vi "Draw_multiple_lines.vi"() -> ()   [LabVIEW 2023]
panel:
  in  "Actualizar":bool
  in  "String":string
  in  "Bobina":T1={"pen"={"Width"=1, "Style"=enum."Solid"}, "color(black)"=0, "fill?(F)"=FALSE, "line endpoints"=[]}
  in  "Resistencia 2":T2={"line endpoints"=[], "pen"={"Width"=1, "Style"=enum."Solid"}, "color(black)"=0, "fill?(F)"=FALSE}
  in  "Fuente":T3={"line endpoints"=[], "pen"={"Width"=1, "Style"=enum."Solid"}, "color(black)"=0, "fill?(F)"=FALSE, "line endpoints 2"=[]}
  in  "Capacitor":T3={"line endpoints"=[], "pen"={"Width"=1, "Style"=enum."Solid"}, "color(black)"=0, "fill?(F)"=FALSE, "line endpoints 2"=[]}
  out "new picture":picture
  in  "stop":bool
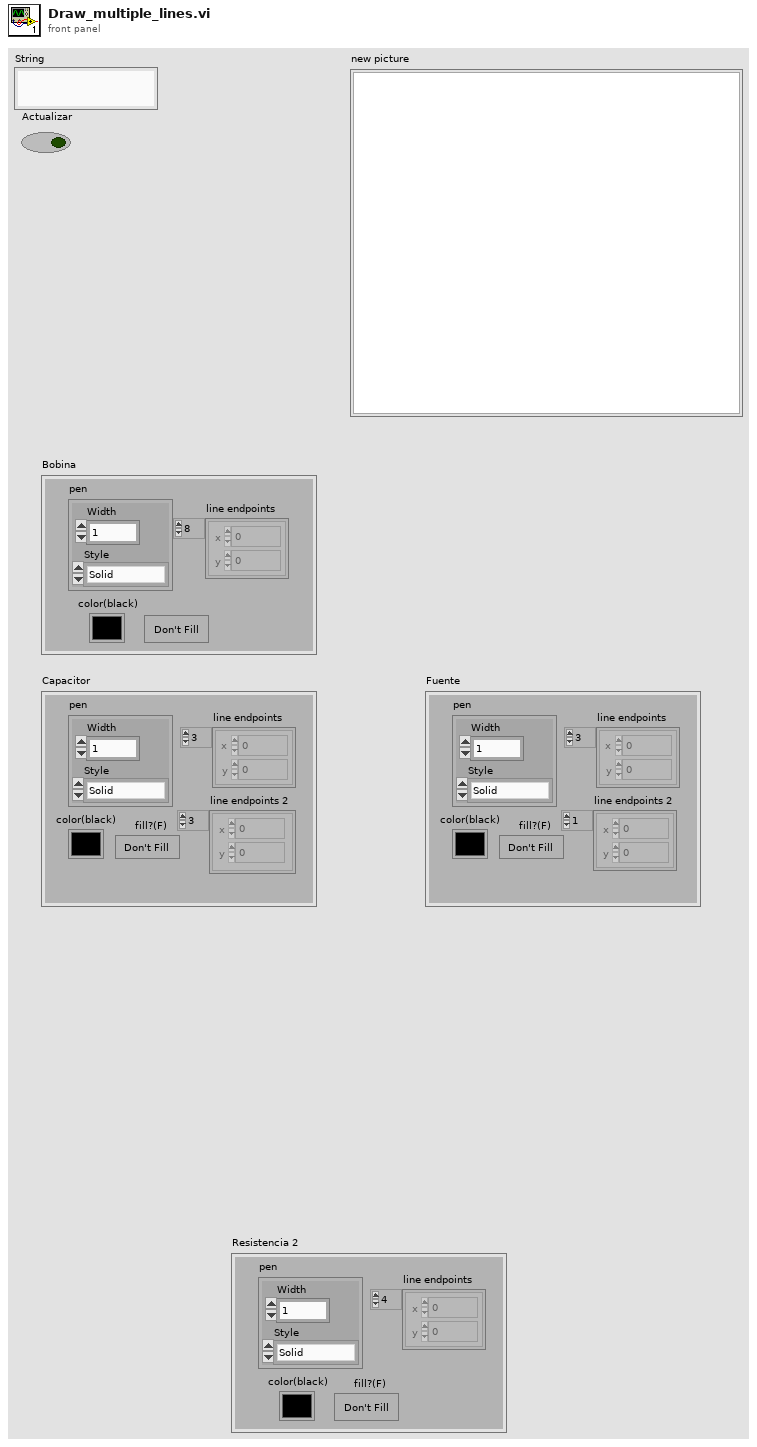
[diagram p1: front panel]
types:
  T1 = cluster{"pen":cluster{"Width":u16, "Style":enum32{"Solid", "Dash", "Dot", "DashDot", "DashDotDot"}}, "color(black)":u32, "fill?(F)":bool, "line endpoints":cluster{"x":i16, "y":i16}[]}
  T2 = cluster{"line endpoints":cluster{"x":i16, "y":i16}[], "pen":cluster{"Width":u16, "Style":enum32{"Solid", "Dash", "Dot", "DashDot", "DashDotDot"}}, "color(black)":u32, "fill?(F)":bool}
  T3 = cluster{"line endpoints":cluster{"x":i16, "y":i16}[], "pen":cluster{"Width":u16, "Style":enum32{"Solid", "Dash", "Dot", "DashDot", "DashDotDot"}}, "color(black)":u32, "fill?(F)":bool, "line endpoints 2":cluster{"x":i16, "y":i16}[]}
  T4 = cluster{"Width":u16, "Style":enum32{"Solid", "Dash", "Dot", "DashDot", "DashDotDot"}}
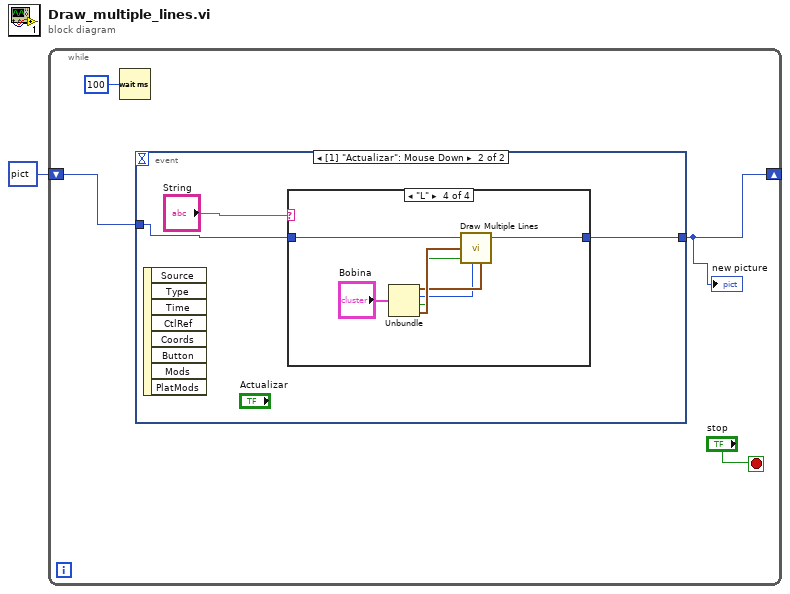
[diagram p0: block diagram]
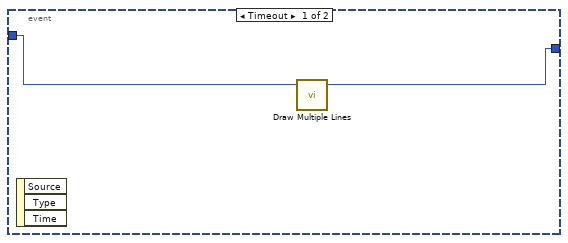
[diagram p2: hidden frame]
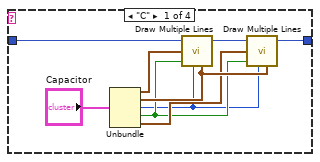
[diagram p3: hidden frame]
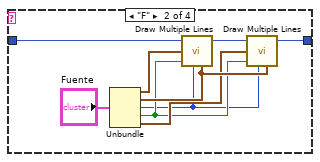
[diagram p4: hidden frame]
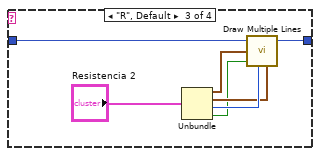
[diagram p5: hidden frame]
diagram:
  n1 = while {
    shift-right: [w2] -> _
    shift-left: picture data[5B] ("picture") -> [w3]
    stop <- "stop" stop-if-true
    n2 = Wait (ms)(milliseconds to wait=u32 100 ("millisecond timer value")) -> ()  [unwired: 1 out]
    n3 = event shown="[1] \"Actualizar\": Mouse Down" {
      selector: _ -> [_ _]
      dyn-events: _ -> [_ _]
      timeout: _ -> [_ _]
      tunnel: w3 -> [w7 w9]
      tunnel: [w6 w8] -> w2
      event Timeout {
        n4 = event-data() -> ()  [unwired: 1 in, 3 out]
        n5 = call <vilib>:"Draw Multiple Lines.vi"("picture"=w7) -> ("new picture"=w6:picture)  [unwired: 8 in]
      }
      event "Actualizar": Mouse Down {
        n6 = event-data() -> ()  [unwired: 1 in, 8 out]
        n7 = case shown="\"L\"" "String" {
          tunnel: w9 -> [w12 w21 w30 w41]
          tunnel: [w11 w20 w29 w40] -> w8
          frame "C" {
            n8 = Unbundle("Capacitor") -> ("line endpoints"=w14:cluster{"x":i16, "y":i16}[], "pen"=w19:T4, "color(black)"=w16:u32, "fill?(F)"=w17:bool, "line endpoints 2"=w18:cluster{"x":i16, "y":i16}[])
            n9 = call <vilib>:"Draw Multiple Lines.vi"("picture"=w12, "line endpoints"=w14, "fill?(F)"=w17, "color(black)"=w16, "pen"=w19) -> ("new picture"=w15:picture)  [unwired: 4 in]
            n10 = call <vilib>:"Draw Multiple Lines.vi"("picture"=w15, "line endpoints"=w18, "fill?(F)"=w17, "color(black)"=w16, "pen"=w19) -> ("new picture"=w11:picture)  [unwired: 4 in]
          }
          frame "F" {
            n11 = Unbundle("Fuente") -> ("line endpoints"=w22:cluster{"x":i16, "y":i16}[], "pen"=w27:T4, "color(black)"=w24:u32, "fill?(F)"=w25:bool, "line endpoints 2"=w26:cluster{"x":i16, "y":i16}[])
            n12 = call <vilib>:"Draw Multiple Lines.vi"("picture"=w21, "line endpoints"=w22, "fill?(F)"=w25, "color(black)"=w24, "pen"=w27) -> ("new picture"=w23:picture)  [unwired: 4 in]
            n13 = call <vilib>:"Draw Multiple Lines.vi"("picture"=w23, "line endpoints"=w26, "fill?(F)"=w25, "color(black)"=w24, "pen"=w27) -> ("new picture"=w20:picture)  [unwired: 4 in]
          }
          frame "R", Default {
            n14 = Unbundle("Resistencia 2") -> ("line endpoints"=w32:cluster{"x":i16, "y":i16}[], "pen"=w34:T4, "color(black)"=w35:u32, "fill?(F)"=w33:bool)
            n15 = call <vilib>:"Draw Multiple Lines.vi"("picture"=w30, "line endpoints"=w32, "fill?(F)"=w33, "color(black)"=w35, "pen"=w34) -> ("new picture"=w29:picture)  [unwired: 4 in]
          }
          frame "L" {
            n16 = Unbundle("Bobina") -> ("pen"=w38:T4, "color(black)"=w37:u32, "fill?(F)"=w36:bool, "line endpoints"=w39:cluster{"x":i16, "y":i16}[])
            n17 = call <vilib>:"Draw Multiple Lines.vi"("picture"=w41, "line endpoints"=w39, "fill?(F)"=w36, "color(black)"=w37, "pen"=w38) -> ("new picture"=w40:picture)  [unwired: 4 in]
          }
        }
      }
    }
    "new picture" <- w2
  }
